vi "Create Licence Key (unidirectional).vi"(8 "error in (no error)":errorcluster, 10 "application name":string, 11 "machine ID":string) -> (0 "error out":errorcluster, 3 "licence key":string)   [LabVIEW 2013]
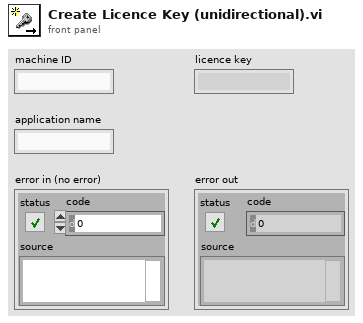
[diagram p1: front panel]
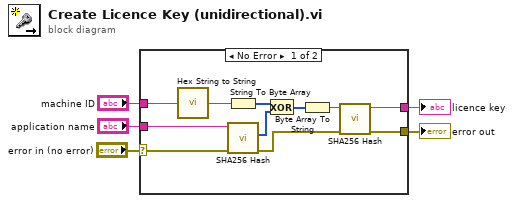
[diagram p0: block diagram]
diagram:
  n1 = case shown="No Error" "error in (no error)" {
    selector: "error in (no error)" -> [w6 w17]
    tunnel: "machine ID" -> [w12 _]
    tunnel: "application name" -> [w10 _]
    tunnel: [w8 _] -> w3
    tunnel: [w7 w17] -> w2
    frame No Error {
      n2 = call "Hex String to String.vi"("hex string"=w12) -> ("string"=w13:string)
      n3 = String To Byte Array(string=w13) -> (unsigned byte array=w11:u8[])
      n4 = call "SHA256 Hash.vi"("error in (no error)"=w6, "string to hash"=w10) -> ("error out"=w9:errorcluster, "hash bytes"=w15:u8[])  [unwired: 7 in, 1 out]
      n5 = Exclusive Or(1:w15, 2:w11) -> (0:w16:u8[])
      n6 = Byte Array To String(unsigned byte array=w16) -> (string=w14:string)
      n7 = call "SHA256 Hash.vi"("error in (no error)"=w9, "string to hash"=w14) -> ("error out"=w7:errorcluster, "hex string hash"=w8:string)  [unwired: 7 in, 1 out]
    }
    frame Error {
    }
  }
  "licence key" <- w3
  "error out" <- w2
